vi "仪器参数转data in.vi"(10 "仪器参数":string, 11 "仪器参数":T2={"测量量程"=0.0, "测量精度"=0.0, "测量间隔"=0.0, "消解温度"=0.0, "消解时长"=0.0, "空白校准时间"=timestamp(0 s since 1904-01-01), "曲线截距"=0.0, "曲线斜率"=0.0, "测量检出限"=0.0, "测量信号值"=0.0, "线性相关系数"=0.0, "二次多项式系数"=0.0, "标样校准时间"=timestamp(0 s since 1904-01-01), "单位"=enum."mg/L"}) -> (3 "data in":T1={"时间标识"=timestamp(0 s since 1904-01-01), "仪器参数"="", "测量量程"=0.0, "测量精度"=0.0, "测量间隔"=0.0, "消解温度"=0.0, "消解时长"=0.0, "空白校准时间"=timestamp(0 s since 1904-01-01), "曲线截距"=0.0, "曲线斜率"=0.0, "测量检出限"=0.0, "测量信号值"=0.0, "线性相关系数"=0.0, "二次多项式系数"=0.0, "标样校准时间"=timestamp(0 s since 1904-01-01), "单位"=enum."mg/L"})   [LabVIEW 2016, in "MB SLAVE.lvlib"]
uses:
  MB SLAVE.lvlib
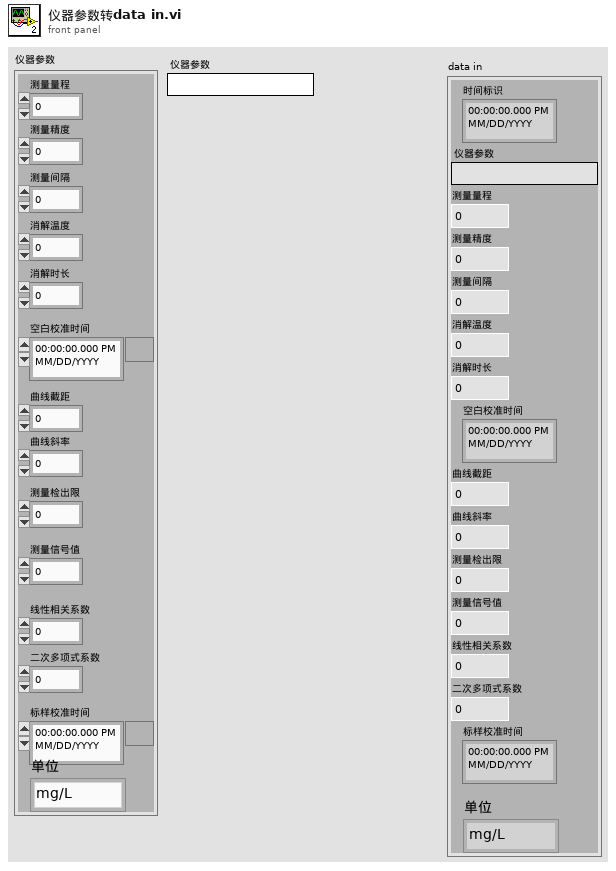
[diagram p1: front panel]
types:
  T1 = cluster{"时间标识":timestamp, "仪器参数":string, "测量量程":dbl, "测量精度":dbl, "测量间隔":dbl, "消解温度":dbl, "消解时长":dbl, "空白校准时间":timestamp, "曲线截距":dbl, "曲线斜率":dbl, "测量检出限":dbl, "测量信号值":dbl, "线性相关系数":dbl, "二次多项式系数":dbl, "标样校准时间":timestamp, "单位":enum16{"ug/L", "mg/L"}}
  T2 = cluster{"测量量程":dbl, "测量精度":dbl, "测量间隔":dbl, "消解温度":dbl, "消解时长":dbl, "空白校准时间":timestamp, "曲线截距":dbl, "曲线斜率":dbl, "测量检出限":dbl, "测量信号值":dbl, "线性相关系数":dbl, "二次多项式系数":dbl, "标样校准时间":timestamp, "单位":enum16{"ug/L", "mg/L"}}
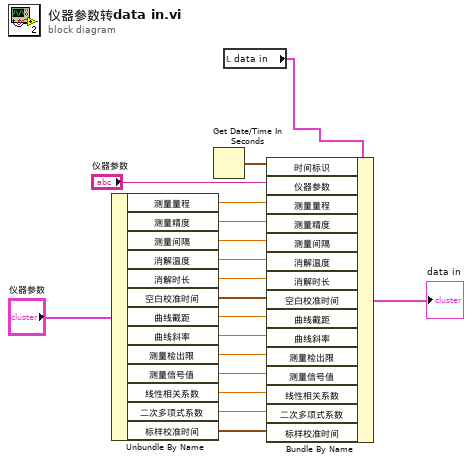
[diagram p0: block diagram]
diagram:
  n1 = Unbundle By Name("仪器参数") -> ("测量量程"=w16:dbl, "测量精度"=w15:dbl, "测量间隔"=w14:dbl, "消解温度"=w13:dbl, "消解时长"=w12:dbl, "空白校准时间"=w11:timestamp, "曲线截距"=w10:dbl, "曲线斜率"=w9:dbl, "测量检出限"=w8:dbl, "测量信号值"=w7:dbl, "线性相关系数"=w6:dbl, "二次多项式系数"=w5:dbl, "标样校准时间"=w4:timestamp)
  n2 = Get Date/Time In Seconds() -> (seconds since 1Jan1904=w18:timestamp)
  n3 = local read "data in"() -> (w1:T1)
  n4 = Bundle By Name(cluster=w1, "时间标识"=w18, "仪器参数"="仪器参数", "测量量程"=w16, "测量精度"=w15, "测量间隔"=w14, "消解温度"=w13, "消解时长"=w12, "空白校准时间"=w11, "曲线截距"=w10, "曲线斜率"=w9, "测量检出限"=w8, "测量信号值"=w7, "线性相关系数"=w6, "二次多项式系数"=w5, "标样校准时间"=w4) -> (→"data in":T1)
